vi "Configure Mask Test.vi"   [LabVIEW 2016, in "Agilent 2000 3000 X-Series.lvlib"]
doc: "Configures the setttings of mast test."
uses:
  Agilent 2000 3000 X-Series.lvlib
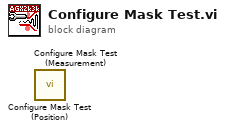
[diagram p0: block diagram]
diagram:
  n1 = call "Configure Mask Test (Position).vi"() -> ()  [unwired: 14 in, 2 out]
  n2 = call "Configure Mask Test (Measurement).vi"() -> ()  [unwired: 14 in, 2 out]
